vi "Close Instruments.vi"(8 "error in":errorcluster, 11 "Manual UI in":refnum<class "Manual UI.lvclass">) -> (0 "error out":errorcluster, 3 "Manual UI out":refnum<class "Manual UI.lvclass">)   [LabVIEW 2023, in "Manual UI.lvlib" / "Manual UI.lvclass"]
uses:
  Project/Manual UI.lvclass
  C:/Users/Public/Documents/Development/builds/Engine/Engine.lvlibp/Project/Engine.lvclass
  Project/Manual UI.lvclass/Manual UI.ctl
  builds/Engine/Actor Framework.lvlibp/1abvi3w/vi.lib/ActorFramework/Message Enqueuer/Message Enqueuer.lvclass
  builds/Engine/Engine.lvlibp/Accessors/Read Report Queue.vi
  builds/Tools/QDMH.lvlibp/Private/Enqueue Unbundled Element.vi
  builds/Tools/QDMH.lvlibp/QDMH.lvclass
  builds/Engine/Actor Framework.lvlibp/1abvi3w/vi.lib/ActorFramework/Stop Msg/Stop Msg.lvclass
  builds/Engine/Engine.lvlibp/Project/Engine.lvclass
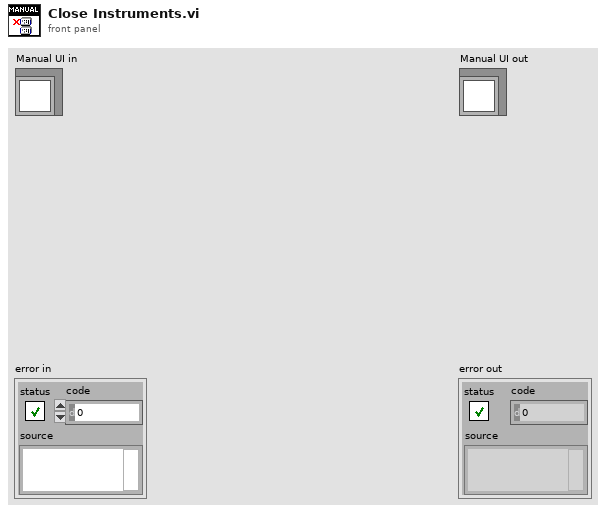
[diagram p1: front panel]
types:
  T1 = cluster{"Identifier":string, "Enqueuer":refnum<class "Message Enqueuer.lvclass">}[]
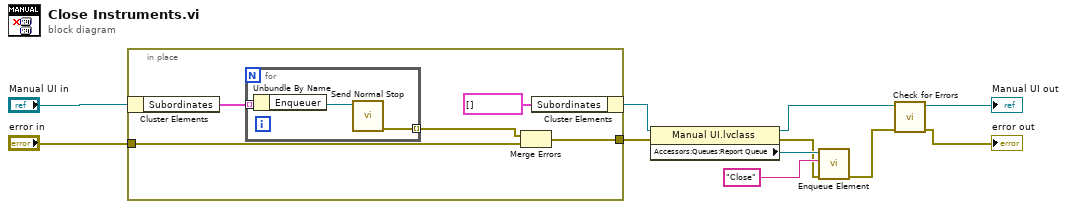
[diagram p0: block diagram]
diagram:
  n1 = in-place {
    in-place-border: "error in" -> [w13]
    in-place-border: [w12] -> w6
    n2 = in-place-cluster #1("Manual UI in") -> ("Subordinates"=w15:T1)
    n3 = for {
      tunnel: w15 -> [w19] mode=indexing
      tunnel: [w17] -> w14 mode=indexing
      n4 = Unbundle By Name(w19) -> ("Enqueuer"=w18:refnum<class "Message Enqueuer.lvclass">)
      n5 = call "Send Normal Stop.vi"("Message Enqueuer"=w18) -> ("error out"=w17:errorcluster)  [unwired: 10 in]
    }
    n6 = Merge Errors(w14, w13) -> (w12:errorcluster)
    n7 = in-place-cluster #1("Subordinates"=T1 []) -> (w7:refnum<class "Manual UI.lvclass">)
  }
  n8 = property class="Manual UI.lvclass"(reference=w7, error in=w6) -> (reference out=w5:refnum<class "Manual UI.lvclass">, error out=w2:errorcluster, "Accessors:Queues:Report Queue"=w4:refnum<class "QDMH.lvclass">)
  n9 = call-poly "Enqueue Element.vi"("error in"=w2, "State"="Close", "QDMH in"=w4) -> ("error out"=w1:errorcluster)  [unwired: 7 in, 1 out]
  n10 = call "Check for Errors.vi"("error in"=w1, "Engine in"=w5) -> ("error out"=→"error out":errorcluster, "Engine out"=→"Manual UI out":refnum<class "Manual UI.lvclass">)  [unwired: 8 in]
